vi "Main.vi"() -> ()   [LabVIEW 2020]
uses:
  <vilib>/Instr/_visa.llb/VISA Find Search Mode.ctl
panel:
  in  "Exit":bool
  in  "Tab Control":T1(tab)
  out "Record Time [s]":ext format="%.2f"
  out "Meas. Periods Recorded":u32
  out "Target Directory":string
  out "Measurement Running":bool
  in  "Stop Recording":bool
  in  "Start Recording":bool
  in  "Measurement Name":string
  in  "Parent Directory":path
  in  "Export Channel 2":bool=TRUE
  in  "Export Channel 1":bool=TRUE
  in  "USB Device Address":string="USB0::0xAE5E::0x0001::00000001::RAW"
  out "Meas. Periods to Process":u32
  out "Data Received [MB]":ext format="%.2f"
  in  "Disconnect":bool
  in  "Connect":bool
  out "Time Domain Plot":waveform(dbl)[](graph)=[{"t0"=timestamp(0 s since 1904-01-01), "dt"=3.90625e-06, "Y"=[]}, {"t0"=timestamp(0 s since 1904-01-01), "dt"=3.90625e-06, "Y"=[]}, {"t0"=timestamp(0 s since 1904-01-01), "dt"=3.90625e-06, "Y"=[]}, {"t0"=timestamp(0 s since 1904-01-01), "dt"=3.90625e-06, "Y"=[]}]
  in  "Remove DC Channel 1":bool=TRUE
  in  "Remove DC Channel 2":bool=TRUE
  in  "Measurement Period [ms]":u16=100 min=5 max=10000 step=5
  out "ENBW [Hz]":dbl
  in  "Weighting Mode":enum16{"Linear", "Exponential"}(ring)=enum."Exponential"
  out "Frequency Resolution [Hz]":dbl min=5.0 max=10000.0 step=5.0
  in  "Number of Averages":dbl=10.0
  out "Averaging Complete":bool
  in  "Restart Averaging":bool
  out "Averages Completed":dbl=1.0
  out "Frequency Domain Plot":cluster{"f0":dbl, "df":dbl, "magnitude":dbl[]}[](graph)=[{"f0"=0.0, "df"=inf, "magnitude"=[]}, {"f0"=0.0, "df"=inf, "magnitude"=[]}, {"f0"=0.0, "df"=inf, "magnitude"=[]}, {"f0"=0.0, "df"=inf, "magnitude"=[]}, {"f0"=0.0, "df"=10.0, "magnitude"=array[12800 elements]}, {"f0"=0.0, "df"=10.0, "magnitude"=array[12800 elements]}]
  in  "Averaging Mode":T2(ring)=enum."RMS averaging"
  in  "Window":u16(ring)=1 items=["Rectangle"=0, "Hanning"=1, "Hamming"=2, "Blackman-Harris"=3, "Exact Blackman"=4, "Blackman"=5, "Flat Top"=6, "Triangle"=30, "Bartlett-Hanning"=31, "Welch"=34, "Kaiser"=60, "Gaussian"=62]
  in  "Spectrum Type":T3(ring)=enum."Amplitude Spectral Density"
  in  "Scaling Channel 2 [dB]":dbl=-20.0
  in  "Scaling Channel 1 [dB]":dbl=-20.0
  in  "Sample Rate [Hz]":u32=256000
  in  "Packet Size [Bytes]":u16=20480
  in  "Packet Length [ms]":u16=5
  in  "Voltage Conversion Factor [V]":dbl=2e-07
  # "NI VISA Data Connection"
  # "File Export"
  # "Status"
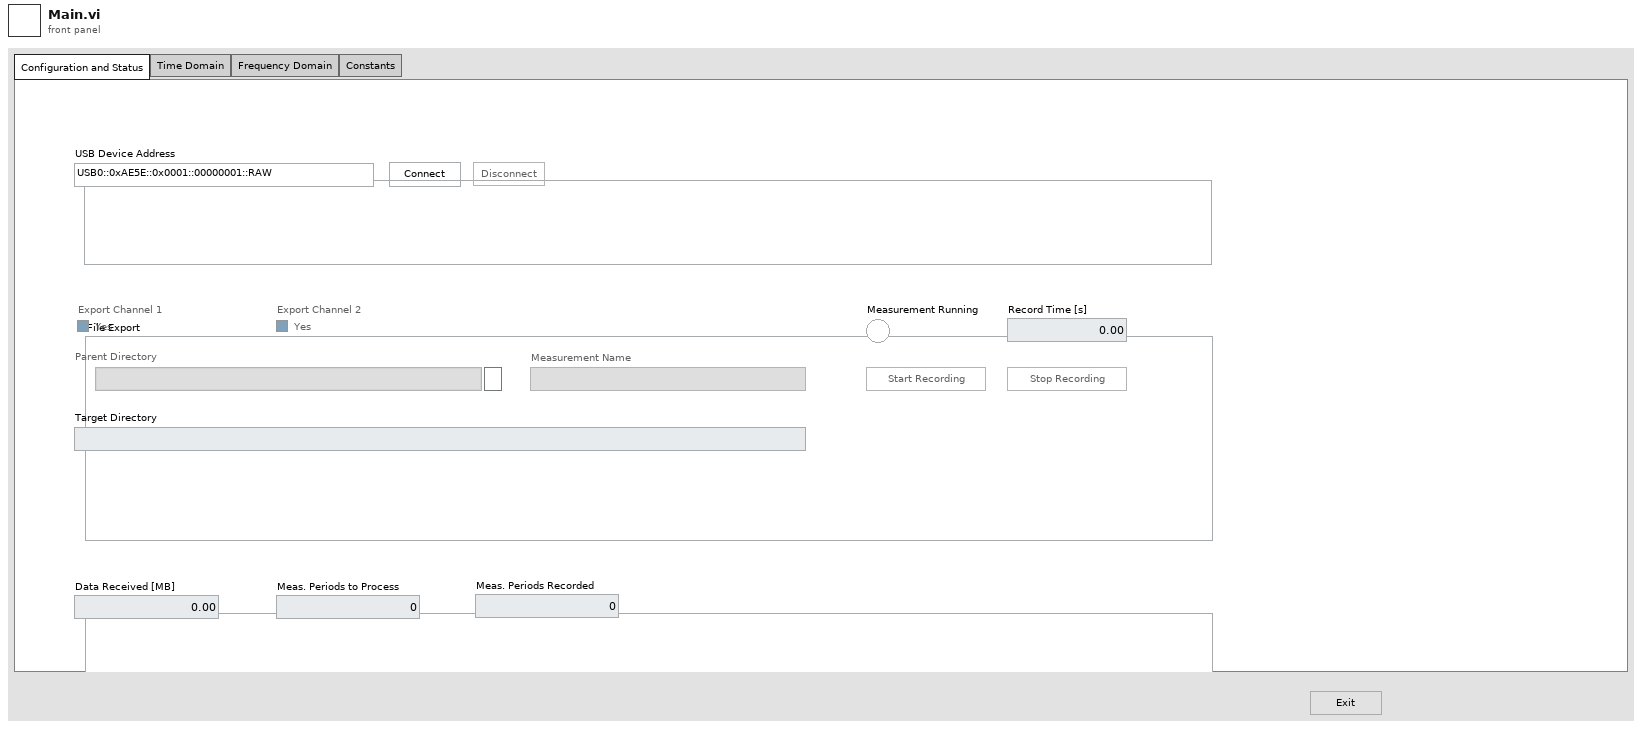
[diagram p1: front panel]
types:
  T1 = enum32{"Configuration and Status", "Time Domain", "Frequency Domain", "Constants"}
  T2 = enum16{"No averaging", "Vector averaging", "RMS averaging", "Peak hold"}
  T3 = enum16{"Amplitude Spectrum", "Amplitude Spectral Density"}
  T4 = enum8{"Enabled", "Disabled", "Disabled and Grayed Out"}
  T5 = typedef "VISA Find Search Mode.ctl" = u32
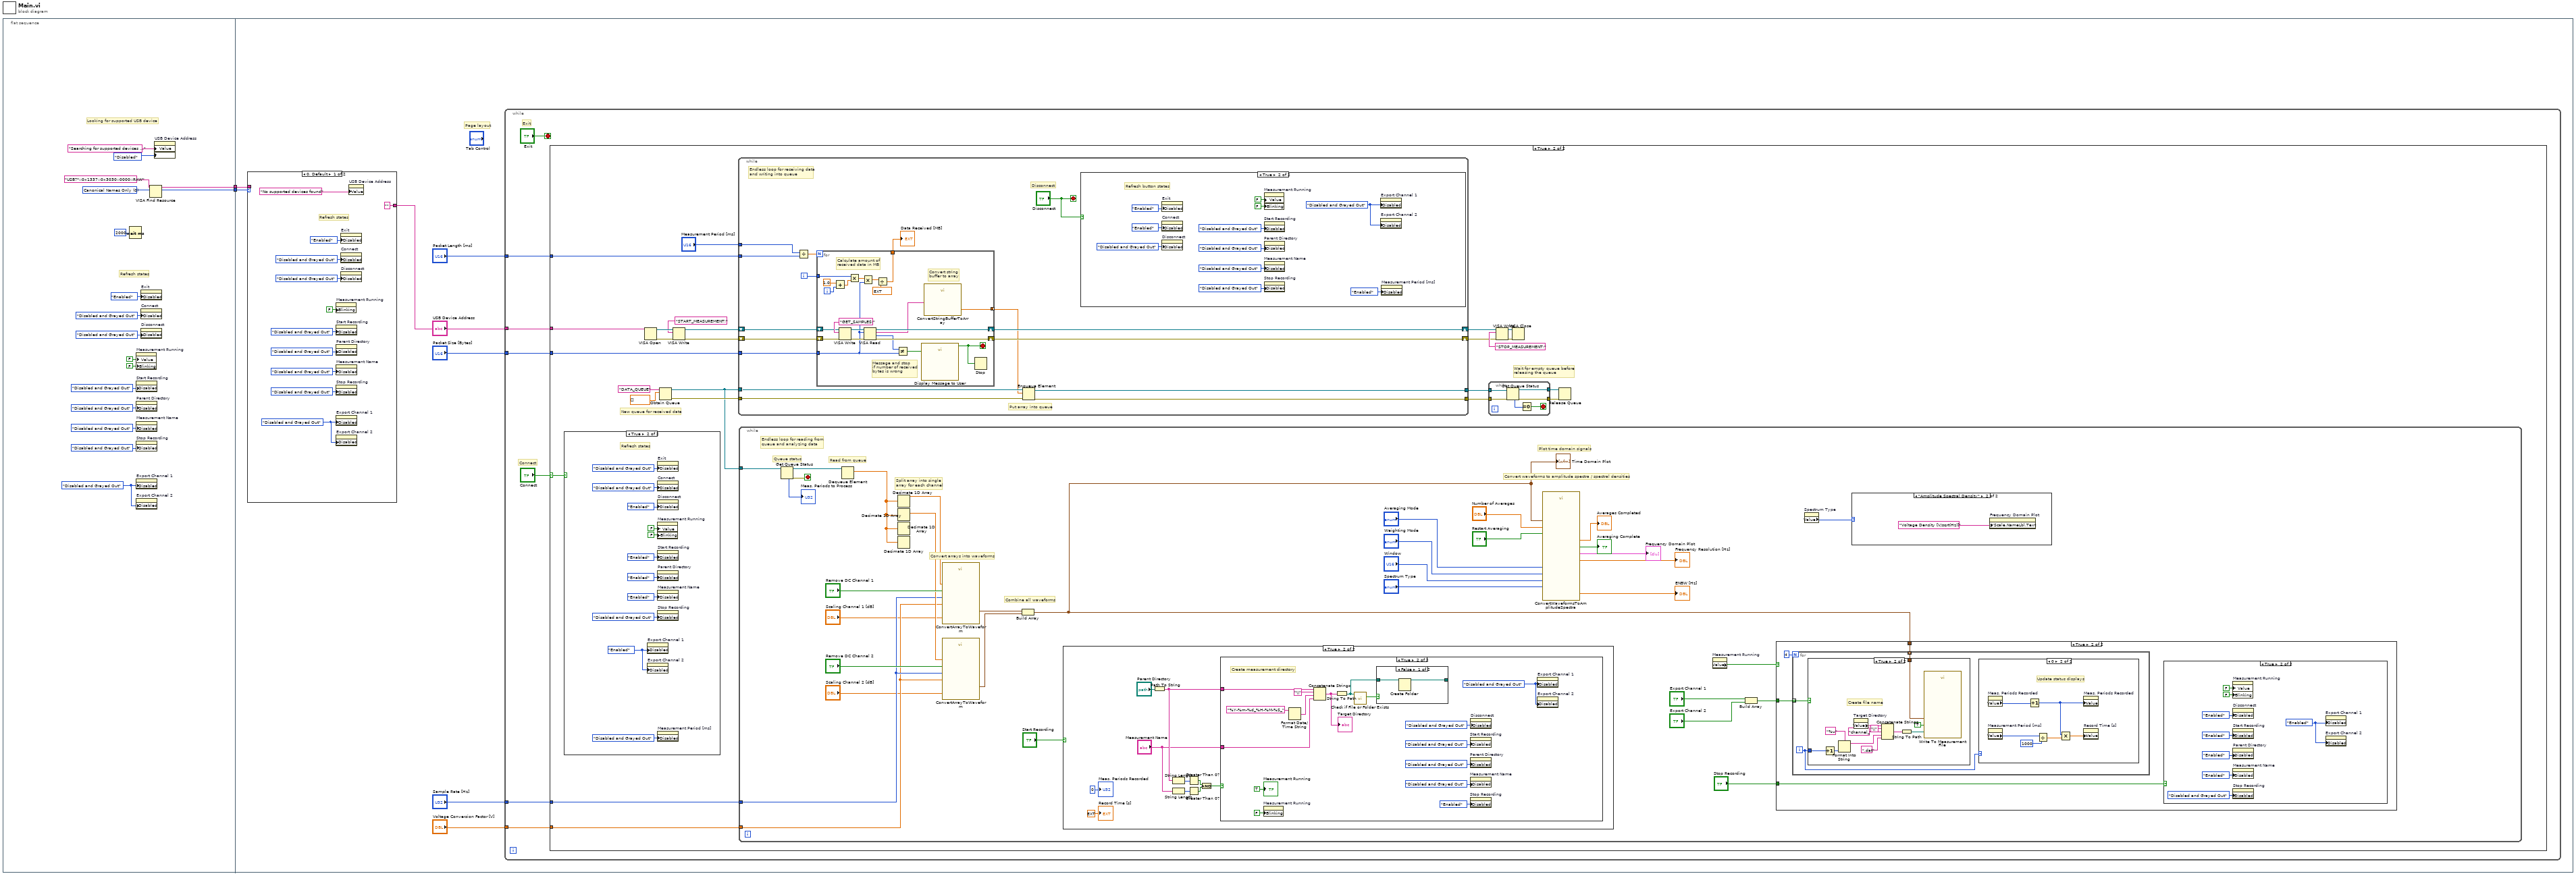
[diagram p0: block diagram]
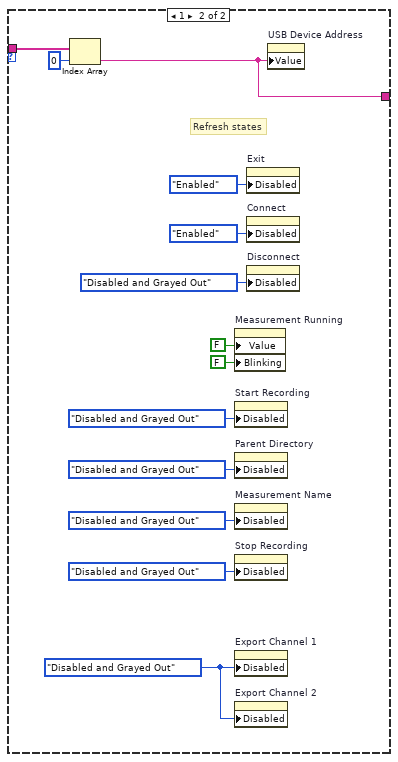
[diagram p2: hidden frame]
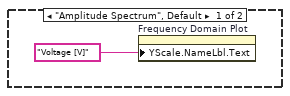
[diagram p4: hidden frame]
diagram:
  n1 = flat-sequence {
    tunnel: [w15] -> w2
    tunnel: [w14] -> w1
    tunnel: w2 -> [w22]
    tunnel: w1 -> [w21]
    frame #0 {
      w3 = T4."Disabled and Grayed Out" ("Disabled")
      w17 = T5 0 items=["Canonical Names Only"=0, "Aliases Only"=2, "Include Matching Aliases"=3, "Include All Aliases"=4] ("Search Mode")
      # "Refresh states"
      # "Looking for supported USB device"
      n2 = Wait (ms)(milliseconds to wait=u32 2000) -> ()  [unwired: 1 out]
      n3 = property on="Measurement Running" class="Bool (strict)"("Value"=FALSE ("Measurement Running"), "Blinking"=FALSE) -> ()  [unwired: 2 in, 2 out]
      n4 = property on="Start Recording" class="Bool"("Disabled"=T4."Disabled and Grayed Out") -> ()  [unwired: 2 in, 2 out]
      n5 = property on="Parent Directory" class="Path"("Disabled"=T4."Disabled and Grayed Out") -> ()  [unwired: 2 in, 2 out]
      n6 = property on="Measurement Name" class="Str"("Disabled"=T4."Disabled and Grayed Out") -> ()  [unwired: 2 in, 2 out]
      n7 = property on="Stop Recording" class="Bool"("Disabled"=T4."Disabled and Grayed Out") -> ()  [unwired: 2 in, 2 out]
      n8 = property on="Export Channel 1" class="Bool (strict)"("Disabled"=w3) -> ()  [unwired: 2 in, 2 out]
      n9 = property on="Export Channel 2" class="Bool (strict)"("Disabled"=w3) -> ()  [unwired: 2 in, 2 out]
      n10 = property on="Exit" class="Bool"("Disabled"=T4."Enabled") -> ()  [unwired: 2 in, 2 out]
      n11 = property on="Connect" class="Bool"("Disabled"=T4."Disabled and Grayed Out") -> ()  [unwired: 2 in, 2 out]
      n12 = property on="Disconnect" class="Bool"("Disabled"=T4."Disabled and Grayed Out") -> ()  [unwired: 2 in, 2 out]
      n13 = VISA Find Resource(10:w17, 11:"USB?*::0x1337::0x3030::0000::RAW" ("expression (\"?*\")")) -> (2:w15:u32, 3:w14:string[])  [unwired: 1 in, 1 out]
      n14 = property on="USB Device Address" class="Str"("Value"="Searching for supported devices ...", "DisabledEnum"=T4."Disabled" ("Disabled")) -> ()  [unwired: 2 in, 2 out]
    }
    frame #1 {
      # "Page layout"
      n15 = case shown="0, Default" w22 {
        tunnel: w21 -> [_ w50]
        tunnel: ["" w45] -> w20
        frame 0, Default {
          w27 = T4."Disabled and Grayed Out" ("Disabled")
          # "Refresh states"
          n16 = property on="Measurement Running" class="Bool (strict)"("Blinking"=FALSE) -> ()  [unwired: 2 in, 2 out]
          n17 = property on="Start Recording" class="Bool"("Disabled"=T4."Disabled and Grayed Out") -> ()  [unwired: 2 in, 2 out]
          n18 = property on="Parent Directory" class="Path"("Disabled"=T4."Disabled and Grayed Out") -> ()  [unwired: 2 in, 2 out]
          n19 = property on="Measurement Name" class="Str"("Disabled"=T4."Disabled and Grayed Out") -> ()  [unwired: 2 in, 2 out]
          n20 = property on="Stop Recording" class="Bool"("Disabled"=T4."Disabled and Grayed Out") -> ()  [unwired: 2 in, 2 out]
          n21 = property on="Export Channel 1" class="Bool (strict)"("Disabled"=w27) -> ()  [unwired: 2 in, 2 out]
          n22 = property on="Export Channel 2" class="Bool (strict)"("Disabled"=w27) -> ()  [unwired: 2 in, 2 out]
          n23 = property on="Exit" class="Bool"("Disabled"=T4."Enabled") -> ()  [unwired: 2 in, 2 out]
          n24 = property on="Connect" class="Bool"("Disabled"=T4."Disabled and Grayed Out") -> ()  [unwired: 2 in, 2 out]
          n25 = property on="Disconnect" class="Bool"("Disabled"=T4."Disabled and Grayed Out") -> ()  [unwired: 2 in, 2 out]
          n26 = property on="USB Device Address" class="Str"("Value"="No supported devices found") -> ()  [unwired: 2 in, 2 out]
        }
        frame 1 {
          w38 = T4."Disabled and Grayed Out" ("Disabled")
          # "Refresh states"
          n27 = Index Array(array=w50, index=0) -> (element=w45:string)
          n28 = property on="Measurement Running" class="Bool (strict)"("Value"=FALSE ("Measurement Running"), "Blinking"=FALSE) -> ()  [unwired: 2 in, 2 out]
          n29 = property on="Start Recording" class="Bool"("Disabled"=T4."Disabled and Grayed Out") -> ()  [unwired: 2 in, 2 out]
          n30 = property on="Parent Directory" class="Path"("Disabled"=T4."Disabled and Grayed Out") -> ()  [unwired: 2 in, 2 out]
          n31 = property on="Measurement Name" class="Str"("Disabled"=T4."Disabled and Grayed Out") -> ()  [unwired: 2 in, 2 out]
          n32 = property on="Stop Recording" class="Bool"("Disabled"=T4."Disabled and Grayed Out") -> ()  [unwired: 2 in, 2 out]
          n33 = property on="Export Channel 1" class="Bool (strict)"("Disabled"=w38) -> ()  [unwired: 2 in, 2 out]
          n34 = property on="Export Channel 2" class="Bool (strict)"("Disabled"=w38) -> ()  [unwired: 2 in, 2 out]
          n35 = property on="Exit" class="Bool"("Disabled"=T4."Enabled") -> ()  [unwired: 2 in, 2 out]
          n36 = property on="Connect" class="Bool"("Disabled"=T4."Enabled") -> ()  [unwired: 2 in, 2 out]
          n37 = property on="Disconnect" class="Bool"("Disabled"=T4."Disabled and Grayed Out") -> ()  [unwired: 2 in, 2 out]
          n38 = property on="USB Device Address" class="Str"("Value"=w45) -> ()  [unwired: 2 in, 2 out]
        }
      }
      n39 = while {
        tunnel: "Packet Size [Bytes]" -> [w56]
        tunnel: w20 -> [w55]
        tunnel: "Packet Length [ms]" -> [w54]
        tunnel: "Sample Rate [Hz]" -> [w53]
        tunnel: "Voltage Conversion Factor [V]" -> [w52]
        stop <- "Exit" stop-if-true
        # "Exit"
        # "Connect"
        n40 = case shown="True" "Connect" {
          selector: "Connect" -> [_ w69]
          tunnel: w55 -> [_ w72]
          tunnel: w56 -> [_ w71]
          tunnel: w54 -> [_ w70]
          tunnel: w53 -> [_ w64]
          tunnel: w52 -> [_ w63]
          frame False {
          }
          frame True {
            # "Wait for empty queue before\nreleasing the queue"
            # "New queue for received data"
            n41 = case shown="True" w69 {
              frame False {
              }
              frame True {
                w188 = T4."Enabled" ("Disabled")
                # "Refresh states"
                n42 = property on="Export Channel 1" class="Bool (strict)"("Disabled"=w188) -> ()  [unwired: 2 in, 2 out]
                n43 = property on="Export Channel 2" class="Bool (strict)"("Disabled"=w188) -> ()  [unwired: 2 in, 2 out]
                n44 = property on="Exit" class="Bool"("Disabled"=T4."Disabled and Grayed Out") -> ()  [unwired: 2 in, 2 out]
                n45 = property on="Connect" class="Bool"("Disabled"=T4."Disabled and Grayed Out") -> ()  [unwired: 2 in, 2 out]
                n46 = property on="Disconnect" class="Bool"("Disabled"=T4."Enabled") -> ()  [unwired: 2 in, 2 out]
                n47 = property on="Measurement Running" class="Bool (strict)"("Value"=FALSE ("Measurement Running"), "Blinking"=FALSE) -> ()  [unwired: 2 in, 2 out]
                n48 = property on="Start Recording" class="Bool"("Disabled"=T4."Enabled") -> ()  [unwired: 2 in, 2 out]
                n49 = property on="Parent Directory" class="Path"("Disabled"=T4."Enabled") -> ()  [unwired: 2 in, 2 out]
                n50 = property on="Measurement Name" class="Str"("Disabled"=T4."Enabled") -> ()  [unwired: 2 in, 2 out]
                n51 = property on="Stop Recording" class="Bool"("Disabled"=T4."Disabled and Grayed Out") -> ()  [unwired: 2 in, 2 out]
                n52 = property on="Measurement Period [ms]" class="DigNum (strict)"("Disabled"=T4."Disabled and Grayed Out") -> ()  [unwired: 2 in, 2 out]
              }
            }
            n53 = VISA Open(VISA resource name=w72) -> (VISA resource name=w81:refnum<visa-resource-name>, error out=w82:errorcluster)  [unwired: 1 in, 3 out]
            n54 = Obtain Queue(name (unnamed)="DATA_QUEUE", element data type=dbl[] [] ("Output Array")) -> (queue out=w65:refnum<queue>, error out=w66:errorcluster)  [unwired: 3 in, 1 out]
            n55 = VISA Write(VISA resource name=w81, write buffer="START_MEASUREMENT;", error in (no error)=w82) -> (VISA resource name out=w79:refnum<visa-resource-name>, error out=w78:errorcluster)  [unwired: 1 out]
            n56 = while {
              shift-right: [w211] -> w77
              shift-left: w79 -> [w213]
              shift-right: [w210] -> w73
              shift-left: w78 -> [w212]
              tunnel: w71 -> [w207]
              tunnel: w70 -> [w208]
              tunnel: w66 -> [w202]
              tunnel: w65 -> [w205]
              tunnel: [w200] -> w62
              tunnel: [w199] -> w61
              tunnel: "Measurement Period [ms]" -> [w198]
              i -> [w201]
              stop <- "Disconnect" stop-if-true
              # "Endless loop for receiving data\nand writing into queue"
              # "Put array into queue"
              # "Disconnect"
              n57 = Divide(x=w198, y=w208) -> (x/y=w209:dbl)
              n58 = for {
                N: w209 -> [_]
                shift-right: [w240] -> w211
                shift-left: w213 -> [w244]
                shift-right: [w239] -> w210
                shift-left: w212 -> [w243]
                tunnel: w201 -> [w237]
                tunnel: w207 -> [w227]
                tunnel: [w233] -> w206
                tunnel: [w229] -> w204 mode=concatenating
                i -> [w230]
                stop <- w225 stop-if-true
                # "Message and stop\nif number of received\nbytes is wrong"
                # "Convert string\nbuffer to array"
                # "Calculate amount of\nreceived data in MB"
                n59 = Add(x=1.0, y=w230) -> (x+y=w232:dbl)
                n60 = VISA Write(VISA resource name=w244, write buffer="GET_SAMPLES;" ("write buffer 2"), error in (no error)=w243) -> (VISA resource name out=w241:refnum<visa-resource-name>, error out=w242:errorcluster)  [unwired: 1 out]
                n61 = Multiply(x=w237, y=w232) -> (x*y=w236:ext)
                n62 = Multiply(x=w236, y=w227) -> (x*y=w235:ext)
                n63 = VISA Read(VISA resource name=w241, byte count=w227, error in (no error)=w242) -> (VISA resource name out=w240:refnum<visa-resource-name>, read buffer=w238:string, return count=w228:u32, error out=w239:errorcluster)
                n64 = Divide(x=w235, y=ext 1000000.0) -> (x/y=w233:ext)
                n65 = Not Equal?(x=w228, y=w227) -> (x != y?=w226:bool)
                n66 = call "Display Message to User"("Enable"=w226) -> ("Exit"=w225:bool)  [unwired: 9 in, 1 out]
                n67 = call "ConvertStringBufferToArray.vi"("Input String Buffer"=w238) -> ("Output Array"=w229:dbl[])  [unwired: 10 in]
                n68 = Stop(stop? (T)=w225) -> ()
              }
              "Data Received [MB]" <- w206
              n69 = Enqueue Element(queue=w205, element=w204, error in (no error)=w202) -> (queue out=w200:refnum<queue>, error out=w199:errorcluster)  [unwired: 1 in, 1 out]
              n70 = case shown="True" "Disconnect" {
                frame False {
                }
                frame True {
                  w215 = T4."Disabled and Grayed Out" ("Disabled")
                  # "Refresh button states"
                  n71 = property on="Exit" class="Bool"("Disabled"=T4."Enabled") -> ()  [unwired: 2 in, 2 out]
                  n72 = property on="Connect" class="Bool"("Disabled"=T4."Enabled") -> ()  [unwired: 2 in, 2 out]
                  n73 = property on="Disconnect" class="Bool"("Disabled"=T4."Disabled and Grayed Out") -> ()  [unwired: 2 in, 2 out]
                  n74 = property on="Measurement Running" class="Bool (strict)"("Value"=FALSE ("Measurement Running"), "Blinking"=FALSE) -> ()  [unwired: 2 in, 2 out]
                  n75 = property on="Start Recording" class="Bool"("Disabled"=T4."Disabled and Grayed Out") -> ()  [unwired: 2 in, 2 out]
                  n76 = property on="Parent Directory" class="Path"("Disabled"=T4."Disabled and Grayed Out") -> ()  [unwired: 2 in, 2 out]
                  n77 = property on="Measurement Name" class="Str"("Disabled"=T4."Disabled and Grayed Out") -> ()  [unwired: 2 in, 2 out]
                  n78 = property on="Stop Recording" class="Bool"("Disabled"=T4."Disabled and Grayed Out") -> ()  [unwired: 2 in, 2 out]
                  n79 = property on="Export Channel 1" class="Bool (strict)"("Disabled"=w215) -> ()  [unwired: 2 in, 2 out]
                  n80 = property on="Export Channel 2" class="Bool (strict)"("Disabled"=w215) -> ()  [unwired: 2 in, 2 out]
                  n81 = property on="Measurement Period [ms]" class="DigNum (strict)"("Disabled"=T4."Enabled") -> ()  [unwired: 2 in, 2 out]
                }
              }
            }
            n82 = while {
              tunnel: w65 -> [w121]
              tunnel: w64 -> [w116]
              tunnel: w63 -> [w115]
              stop <- w110 stop-if-true
              # "Combine all waveforms"
              # "Convert waveforms to amplitude spectra / spectral densities"
              # "Endless loop for reading from\nqueue and analyzing data"
              # "Plot time domain signals"
              # "Convert arrays into waveforms"
              # "Split array into single\narray for each channel"
              # "Read from queue"
              # "Queue status"
              n83 = Get Queue Status(queue=w121) -> (queue out=w111:refnum<queue>, error out=w110:errorcluster, # elements in queue=→"Meas. Periods to Process":i32)  [unwired: 2 in, 5 out]
              n84 = Dequeue Element(queue=w111) -> (element=w100:dbl[])  [unwired: 2 in, 3 out]
              n85 = Decimate 1D Array(w100) -> (w118:dbl[])  [unwired: 3 out]
              n86 = Decimate 1D Array(w100) -> (w117:dbl[])  [unwired: 3 out]
              n87 = Decimate 1D Array(w100) -> ()  [unwired: 4 out]
              n88 = Decimate 1D Array(w100) -> ()  [unwired: 4 out]
              n89 = call "ConvertArrayToWaveform.vi"("Scaling [dB]"="Scaling Channel 1 [dB]", "Remove DC"="Remove DC Channel 1", "Input Array"=w118, "Voltage Conversion Factor [V]"=w115, "Sample Rate [Hz]"=w116) -> ("Output Waveform"=w109:waveform(dbl))  [unwired: 6 in]
              n90 = call "ConvertArrayToWaveform.vi"("Scaling [dB]"="Scaling Channel 2 [dB]", "Remove DC"="Remove DC Channel 2", "Input Array"=w117, "Voltage Conversion Factor [V]"=w115, "Sample Rate [Hz]"=w116) -> ("Output Waveform"=w108:waveform(dbl))  [unwired: 6 in]
              n91 = Build Array(w109, w108) -> (w98:waveform(dbl)[])
              "Time Domain Plot" <- w98
              n92 = case shown="True" "Start Recording" {
                frame False {
                }
                frame True {
                  n93 = Path To String(path="Parent Directory") -> (string=w166:string)
                  n94 = String Length(string=w166) -> (length=w164:i32)
                  n95 = String Length(string="Measurement Name") -> (length=w163:i32)
                  n96 = Greater Than 0?(x=w164) -> (x > 0?=w162:bool)
                  n97 = Greater Than 0?(x=w163) -> (x > 0?=w161:bool)
                  n98 = And(x=w162, y=w161) -> (x .and. y?=w160:bool)
                  n99 = case shown="True" w160 {
                    tunnel: w166 -> [_ w183]
                    tunnel: "Measurement Name" -> [_ w177]
                    frame False {
                    }
                    frame True {
                      w168 = T4."Disabled and Grayed Out" ("Disabled")
                      # "Create measurement directory"
                      n100 = property on="Measurement Running" class="Bool (strict)"("Blinking"=FALSE) -> ()  [unwired: 2 in, 2 out]
                      n101 = Format Date/Time String(time format string (%c)="%Y-%m-%d_%H-%M-%S_") -> (date/time string=w178:string)  [unwired: 2 in]
                      n102 = Concatenate Strings(w183, "\\" ("string"), w178, w177) -> (w170:string)
                      "Target Directory" <- w170
                      n103 = String To Path(string=w170) -> (path=w180:path)
                      n104 = call <vilib>:"Check if File or Folder Exists.vi"("path"=w180) -> ("file or folder exists?"=w181:bool)  [unwired: 8 in, 2 out]
                      n105 = case shown="False" w181 {
                        tunnel: w180 -> [w185 w186]
                        tunnel: [w184 w186] -> _
                        frame False {
                          n106 = Create Folder(path (use dialog)=w185) -> (created path=w184:path)  [unwired: 2 in, 2 out]
                        }
                        frame True {
                        }
                      }
                      n107 = property on="Start Recording" class="Bool"("Disabled"=T4."Disabled and Grayed Out") -> ()  [unwired: 2 in, 2 out]
                      n108 = property on="Parent Directory" class="Path"("Disabled"=T4."Disabled and Grayed Out") -> ()  [unwired: 2 in, 2 out]
                      n109 = property on="Measurement Name" class="Str"("Disabled"=T4."Disabled and Grayed Out") -> ()  [unwired: 2 in, 2 out]
                      n110 = property on="Stop Recording" class="Bool"("Disabled"=T4."Enabled") -> ()  [unwired: 2 in, 2 out]
                      n111 = property on="Disconnect" class="Bool"("Disabled"=T4."Disabled and Grayed Out") -> ()  [unwired: 2 in, 2 out]
                      n112 = property on="Export Channel 1" class="Bool (strict)"("Disabled"=w168) -> ()  [unwired: 2 in, 2 out]
                      n113 = property on="Export Channel 2" class="Bool (strict)"("Disabled"=w168) -> ()  [unwired: 2 in, 2 out]
                      "Measurement Running" <- TRUE
                    }
                  }
                  "Meas. Periods Recorded" <- u32 0 ("Meas. Periods Recorded")
                  "Record Time [s]" <- ext 0.0 ("Record Time [s]")
                }
              }
              n114 = call "ConvertWaveformsToAmplitudeSpectra.vi"("Averaging Mode"="Averaging Mode", "Number of Averages"="Number of Averages", "Weighting Mode"="Weighting Mode", "Export Mode"="Spectrum Type", "Waveforms"=w98, "Window"="Window", "Restart Averaging"="Restart Averaging") -> ("Frequency Resolution [Hz]"=→"Frequency Resolution [Hz]":dbl, "Amplitude Spectral Density"=→"Frequency Domain Plot":cluster{"f0":dbl, "df":dbl, "magnitude":dbl[]}[], "Averages Completed"=→"Averages Completed":dbl, "Averaging Done"=→"Averaging Complete":bool, "ENBW [Hz]"=→"ENBW [Hz]":dbl)
              n115 = property on="Measurement Running" class="Bool (strict)"() -> ("Value"=w104:bool)  [unwired: 2 in, 2 out]
              n116 = Build Array("Export Channel 1", "Export Channel 2") -> (w102:bool[])
              n117 = case shown="True" w104 {
                tunnel: "Stop Recording" -> [_ w128]
                tunnel: w102 -> [_ w127]
                tunnel: w98 -> [_ w125]
                frame False {
                }
                frame True {
                  n118 = for {
                    N: 4 -> [_]
                    tunnel: w127 -> [w131] mode=indexing
                    tunnel: w125 -> [w130] mode=indexing
                    i -> [w129]
                    n119 = case shown="True" w131 {
                      tunnel: w129 -> [_ w145]
                      tunnel: w130 -> [_ w139]
                      frame False {
                      }
                      frame True {
                        # "Create file name"
                        n120 = Increment(x=w145) -> (x+1=w144:i32)
                        n121 = Format Into String(format string="%u", w144) -> (resulting string=w142:string)  [unwired: 2 in, 1 out]
                        n122 = property on="Target Directory" class="Str"() -> ("Value"=w147:string)  [unwired: 2 in, 2 out]
                        n123 = Concatenate Strings(w147, "\\" ("string"), "channel_" ("string"), w142, ".dat" ("string")) -> (w146:string)
                        n124 = String To Path(string=w146) -> (path=w140:path)
                        n125 = call "Write To Measurement File"("Signals"=w139, "Enable"=TRUE, "Filename"=w140) -> ()  [unwired: 14 in, 3 out]
                      }
                    }
                    n126 = case shown="0" w129 {
                      frame -1, Default {
                      }
                      frame 0 {
                        # "Update status displays"
                        n127 = property on="Meas. Periods Recorded" class="DigNum (strict)"() -> ("Value"=w134:u32)  [unwired: 2 in, 2 out]
                        n128 = property on="Measurement Period [ms]" class="DigNum (strict)"() -> ("Value"=w136:u16)  [unwired: 2 in, 2 out]
                        n129 = Increment(x=w134) -> (x+1=w133:u32)
                        n130 = Divide(x=w136, y=u16 1000) -> (x/y=w137:dbl)
                        n131 = Multiply(x=w133, y=w137) -> (x*y=w132:dbl)
                        n132 = property on="Meas. Periods Recorded" class="DigNum (strict)"("Value"=w133) -> ()  [unwired: 2 in, 2 out]
                        n133 = property on="Record Time [s]" class="DigNum (strict)"("Value"=w132) -> ()  [unwired: 2 in, 2 out]
                      }
                    }
                  }
                  n134 = case shown="True" w128 {
                    frame False {
                    }
                    frame True {
                      w150 = T4."Enabled" ("Disabled")
                      n135 = property on="Measurement Running" class="Bool (strict)"("Value"=FALSE ("Measurement Running"), "Blinking"=FALSE) -> ()  [unwired: 2 in, 2 out]
                      n136 = property on="Disconnect" class="Bool"("Disabled"=T4."Enabled") -> ()  [unwired: 2 in, 2 out]
                      n137 = property on="Start Recording" class="Bool"("Disabled"=T4."Enabled") -> ()  [unwired: 2 in, 2 out]
                      n138 = property on="Parent Directory" class="Path"("Disabled"=T4."Enabled") -> ()  [unwired: 2 in, 2 out]
                      n139 = property on="Measurement Name" class="Str"("Disabled"=T4."Enabled") -> ()  [unwired: 2 in, 2 out]
                      n140 = property on="Stop Recording" class="Bool"("Disabled"=T4."Disabled and Grayed Out") -> ()  [unwired: 2 in, 2 out]
                      n141 = property on="Export Channel 1" class="Bool (strict)"("Disabled"=w150) -> ()  [unwired: 2 in, 2 out]
                      n142 = property on="Export Channel 2" class="Bool (strict)"("Disabled"=w150) -> ()  [unwired: 2 in, 2 out]
                    }
                  }
                }
              }
              n143 = property on="Spectrum Type" class="Enum (strict)"() -> ("Value"=w91:T3)  [unwired: 2 in, 2 out]
              n144 = case shown="\"Amplitude Spectral Density\"" w91 {
                frame "Amplitude Spectrum", Default {
                  n145 = property on="Frequency Domain Plot" class="WFGraph (strict)"("YScale.NameLbl.Text"="Voltage [V]" ("Y Scale.Name Label.Text")) -> ()  [unwired: 2 in, 2 out]
                }
                frame "Amplitude Spectral Density" {
                  n146 = property on="Frequency Domain Plot" class="WFGraph (strict)"("YScale.NameLbl.Text"="Voltage Density [V/sqrt(Hz)]" ("Y Scale.Name Label.Text")) -> ()  [unwired: 2 in, 2 out]
                }
              }
            }
            n147 = while {
              tunnel: w62 -> [w88]
              tunnel: w61 -> [w87]
              tunnel: [w84] -> w60
              tunnel: [w83] -> w59
              stop <- w86 stop-if-true
              n148 = Get Queue Status(queue=w88, error in (no error)=w87) -> (queue out=w84:refnum<queue>, error out=w83:errorcluster, # elements in queue=w85:i32)  [unwired: 1 in, 5 out]
              n149 = Equal To 0?(x=w85) -> (x = 0?=w86:bool)
            }
            n150 = VISA Write(VISA resource name=w77, write buffer="STOP_MEASUREMENT;" ("write buffer 3"), error in (no error)=w73) -> (VISA resource name out=w75:refnum<visa-resource-name>, error out=w76:errorcluster)  [unwired: 1 out]
            n151 = VISA Close(VISA resource name=w75, error in (no error)=w76) -> ()  [unwired: 1 out]
            n152 = Release Queue(queue=w60, error in (no error)=w59) -> ()  [unwired: 1 in, 3 out]
          }
        }
      }
    }
  }
